vi "EventstoGraph (SubVI).vi"(6 "Numerisch 2":dbl, 7 "Array 3":dbl[](array[numeric]), 9 "Numerisch":dbl, 10 "Array (Eingang)":dbl[][](array[numeric]), 11 "Numerisch 3":dbl) -> (3 "Array (Ausgang)":dbl[][](array[numeric]))   [LabVIEW 2024]
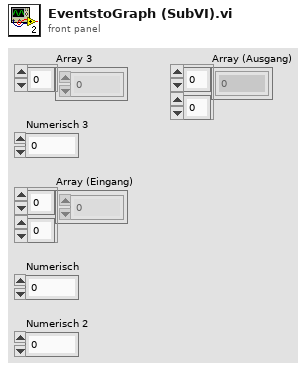
[diagram p1: front panel]
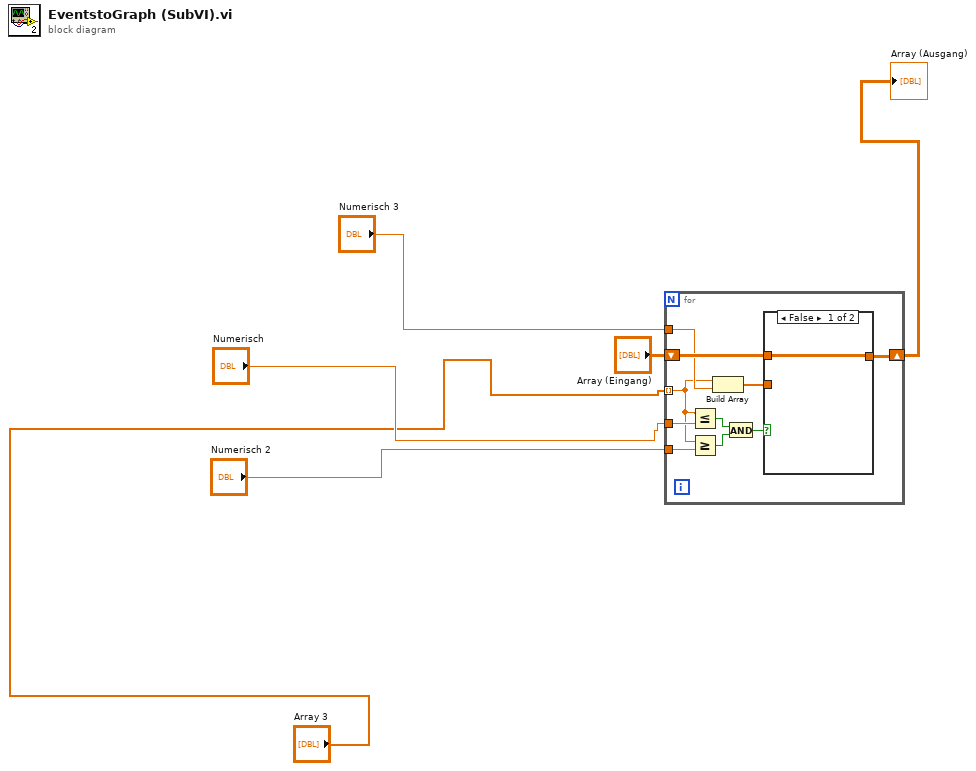
[diagram p0: block diagram]
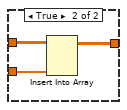
[diagram p2: hidden frame]
diagram:
  n1 = for {
    tunnel: "Numerisch 3" -> [w8]
    tunnel: "Array 3" -> [w7] mode=indexing
    tunnel: "Numerisch 2" -> [w16]
    tunnel: "Numerisch" -> [w15]
    shift-right: [w11] -> w6
    shift-left: "Array (Eingang)" -> [w12]
    n2 = Less Or Equal?(x=w7, y=w15) -> (x <= y?=w13:bool)
    n3 = Greater Or Equal?(x=w7, y=w16) -> (x >= y?=w14:bool)
    n4 = Build Array(w7, w8) -> (w9:dbl[])
    n5 = And(x=w13, y=w14) -> (x .and. y?=w10:bool)
    n6 = case shown="False" w10 {
      tunnel: w12 -> [w17 w20]
      tunnel: [w17 w19] -> w11
      tunnel: w9 -> [_ w18]
      frame False {
      }
      frame True {
        n7 = Insert Into Array(array=w20, new element=w18) -> (w19:dbl[][])  [unwired: 2 in]
      }
    }
  }
  "Array (Ausgang)" <- w6
